vi "CreateError.vi"(5 "MergeErrors":bool, 6 "AdditionalText":string, 7 "Data":variant, 8 "ErrorIn":errorcluster caption="Error In", 9 "Text":string, 10 "ErrorCode":i32) -> (0 "ErrorOut":errorcluster caption="Error Out")   [LabVIEW 2018, in "ErrorCreationExecution.lvclass"]
uses:
  ErrorCreationExecution.lvclass
  ErrorCreationTypes/ErrorCreationMGI/ErrorCreationMGI.lvclass
  C:/Localdata/Projects/TriekselSoft/CustomErrorCreator/Source/ErrorCreationExecution/ErrorCreationExecution.lvclass
  ErrorCreationType.vi
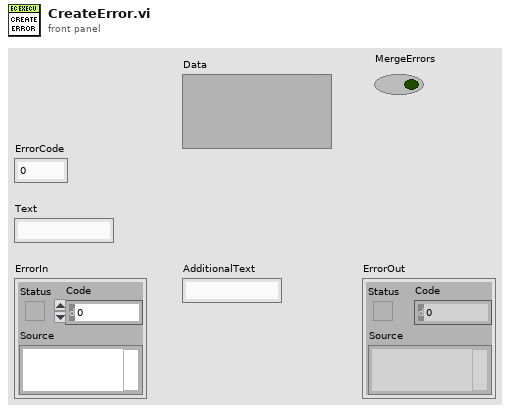
[diagram p1: front panel]
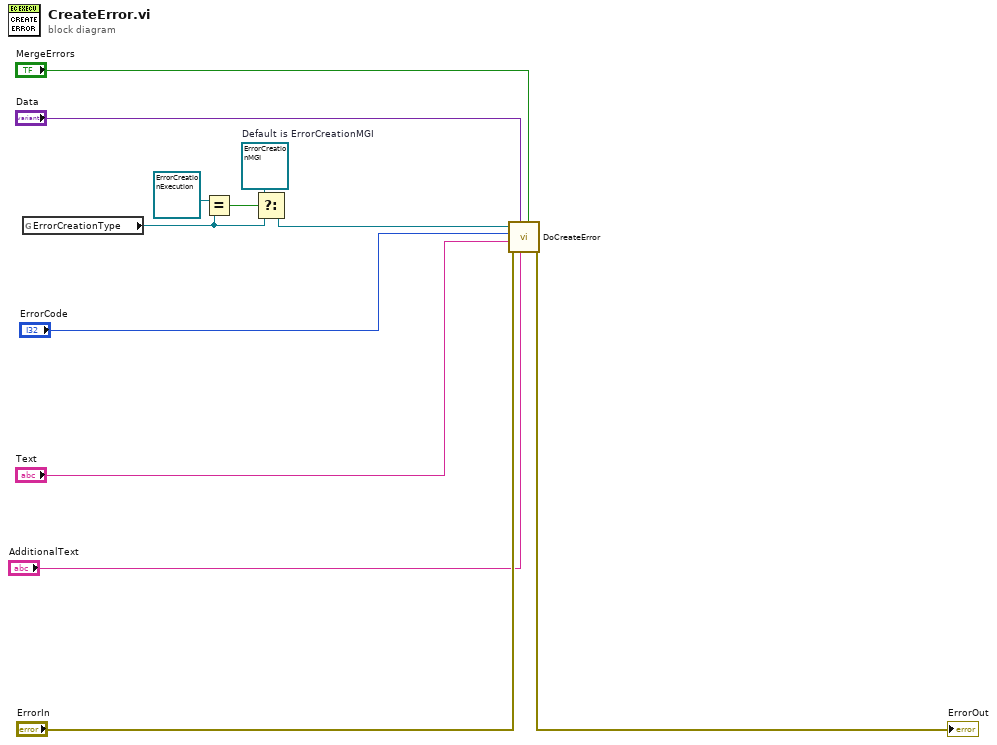
[diagram p0: block diagram]
diagram:
  w2 = refnum<class "ErrorCreationMGI.lvclass"> refnum  # Default is ErrorCreationMGI
  n1 = global read "ErrorCreationType.vi" "ErrorCreationType"() -> (w4:refnum<class "ErrorCreationExecution.lvclass">)
  n2 = Equal?(x=refnum<class "ErrorCreationExecution.lvclass"> refnum ("ErrorCreationExecution"), y=w4) -> (x = y?=w5:bool)
  n3 = Select(t=w2, s=w5, f=w4) -> (s? t:f=w3:refnum<class "ErrorCreationExecution.lvclass">)
  n4 = call-dynamic "DoCreateError.vi"("MergeErrors"="MergeErrors", "AdditionalText"="AdditionalText", "Data"="Data", "ErrorIn"="ErrorIn", "Text"="Text", "ErrorCode"="ErrorCode", "ObjectIn"=w3) -> ("ErrorOut"=→"ErrorOut":errorcluster)  [unwired: 3 in, 1 out]
